vi "Config GUI - Section Header Selected.vi"(7 "User VI Owner Status":T1, 8 "error in":errorcluster, 9 "GUI Objects":T2, 10 "SCL Value (Selected Row Index)":i32) -> (0 "error out":errorcluster)   [LabVIEW 2021]
doc: "Disables some of the GUI objects when a section header is selected in the SCL (because a section header is not a template or VI that a new VI can be created from, so need to disable objects such as the \"Create\" button, etc).\n\nEnables all objects when a non-header item is selected in the SCL list, because a non-header implies a valid CTL or VI being selected."
uses:
  GUI Objects (cluster).ctl
  Owner Status (enum).ctl
panel:
  # "Development\ncontrols/indicators useful for development and testing, but which are not outputs of the VI"
  # "Input\nInputs to the VI"
  # "Output\nOutputs of the VI"
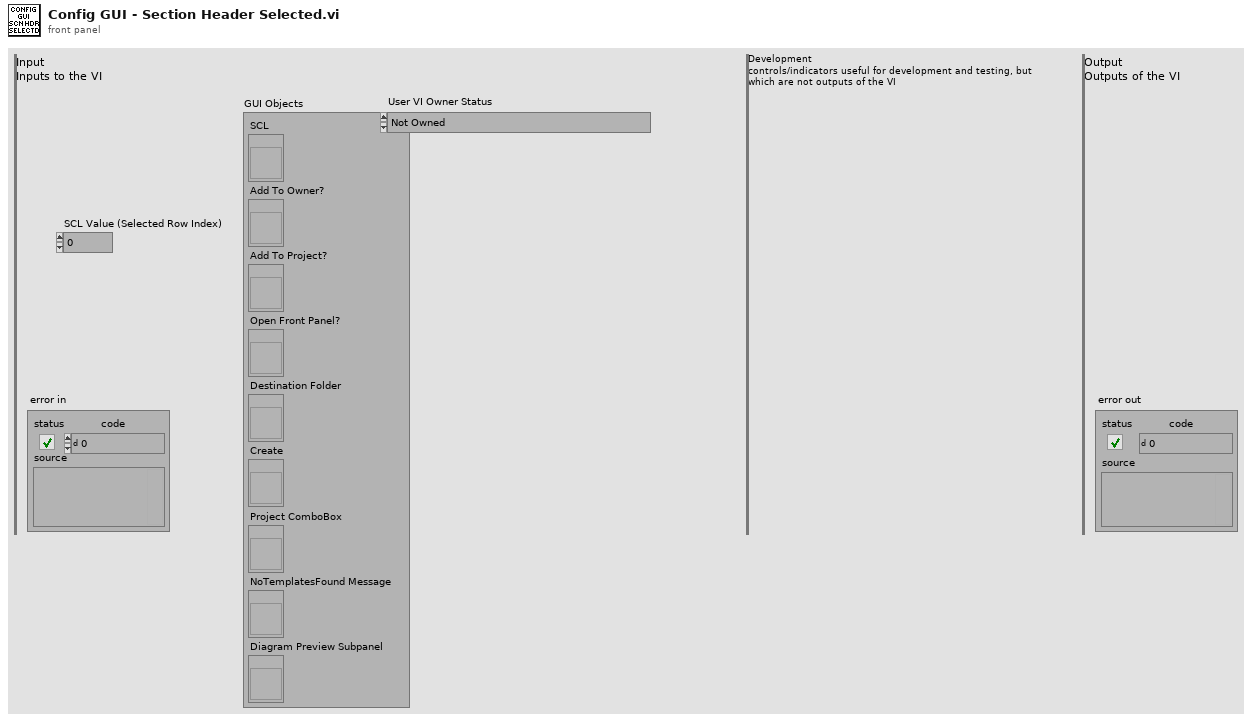
[diagram p1: front panel]
types:
  T1 = typedef "Owner Status (enum).ctl" = enum16{"Not Owned", "Owned by Library (lvlib)", "Owned by Class (lvclass)"}
  T2 = typedef "GUI Objects (cluster).ctl" = cluster{"SCL":refnum<vi>, "Add To Owner?":refnum<vi>, "Add To Project?":refnum<vi>, "Open Front Panel?":refnum<vi>, "Destination Folder":refnum<vi>, "Create":refnum<vi>, "Project ComboBox":refnum<vi>, "NoTemplatesFound Message":refnum<vi>, "Diagram Preview Subpanel":refnum<vi>}
  T3 = enum8{"Enabled", "Disabled", "Disabled and Grayed Out"}
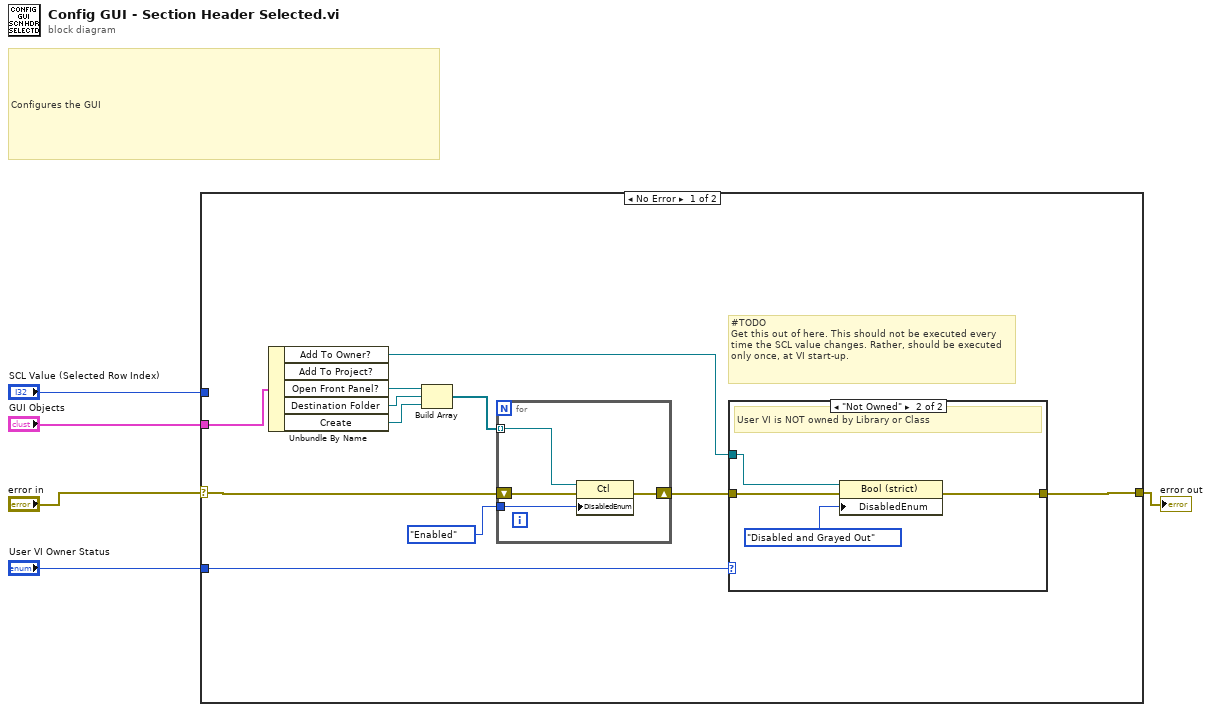
[diagram p0: block diagram]
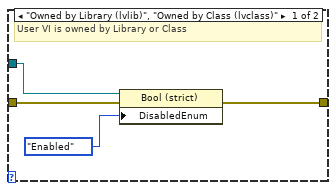
[diagram p2: hidden frame]
diagram:
  # "Configures the GUI"
  n1 = case shown="No Error" "error in" {
    selector: "error in" -> [w16 w29]
    tunnel: [w15 w29] -> w4
    tunnel: "SCL Value (Selected Row Index)" -> [_ _]
    tunnel: "GUI Objects" -> [w14 _]
    tunnel: "User VI Owner Status" -> [w13 _]
    frame No Error {
      # "#TODO\nGet this out of here. This should not be executed every time the SCL value changes. Rather, should be executed only once, at VI start-up."
      n2 = Unbundle By Name(w14) -> ("Add To Owner?"=w7:refnum<vi>, "Open Front Panel?"=w12:refnum<vi>, "Destination Folder"=w9:refnum<vi>, "Create"=w10:refnum<vi>)  [unwired: 1 out]
      n3 = Build Array(w12, w9, w10) -> (w11:refnum<vi>[])
      n4 = for {
        shift-right: [w27] -> w6
        shift-left: w16 -> [w28]
        tunnel: w11 -> [w26] mode=indexing
        tunnel: T3."Enabled" ("Disabled") -> [w25]
        n5 = property class="Ctl"(reference=w26, error in=w28, "DisabledEnum"=w25) -> (error out=w27:errorcluster)  [unwired: 1 out]
      }
      n6 = case shown="\"Not Owned\"" w13 {
        tunnel: w7 -> [w18 w22]
        tunnel: w6 -> [w20 w24]
        tunnel: [w17 w21] -> w15
        frame "Owned by Library (lvlib)", "Owned by Class (lvclass)" {
          # "User VI is owned by Library or Class"
          n7 = property class="Bool (strict)"(reference=w18, error in=w20, "DisabledEnum"=T3."Enabled" ("Disabled")) -> (error out=w17:errorcluster)  [unwired: 1 out]
        }
        frame "Not Owned" {
          # "User VI is NOT owned by Library or Class"
          n8 = property class="Bool (strict)"(reference=w22, error in=w24, "DisabledEnum"=T3."Disabled and Grayed Out" ("Disabled")) -> (error out=w21:errorcluster)  [unwired: 1 out]
        }
      }
    }
    frame Error {
    }
  }
  "error out" <- w4
